vi "NI 9223 User-Controlled IO Sampling (FPGA).vi"() -> ()   [LabVIEW 2012]
doc: "This VI reads a user-defined number of points of calibrated data from all 4 channels of a NI 9223 at the specificed rate using the User-Controlled I/O Sampling API."
uses:
  <vilib>/rvi/eio/common/nirviEmuClasses.ctl
  <vilib>/rvi/eio/common/nirviEmuTemplateMethod_errors.vi
  <vilib>/rvi/Emulation/niFpgaSctlEmulationGetInTimedLoop.vi
  <vilib>/rvi/Emulation/niFpgaSctlEmulationGlobalWrite.vi
  <vilib>/rvi/interface/RandomDataEmulation/nirviRandomDataFPGAFIFO.vi
  <vilib>/rvi/interface/RandomDataEmulation/niFpgaRandomDataHandleErrors.vi
  <vilib>/eio/EIOGrowableMethodNode/genericMethod/EIOGrowableMethodNode.xnode
  <vilib>/rvi/eio/nirviEIOMethodImplementation/nirviEIOMethodImplementation.xnode
  <vilib>/rvi/eio/nirviErrorMerge/nirviErrorMerge.xnode
  <vilib>/rvi/DataTransferAndStorage/Container/XNode/niFpgaContainer.xnode
  <vilib>/rvi/interface/RandomDataEmulation/nirviRandomDataFpgaReadWriteTemplate.vi
panel:
  out "Error":bool
  in  "Number of Samples":u32=5000
  out "Error Out":errorcluster
  out "Stopped":bool
  out "Timed Out":bool
  out "Sample Gated":bool
  out "Overwrite":bool
  in  "Sample Period (uSec)":u32=1
  # "For instructions, and select Help>>Show Context Help and hover over the icon."
  # "Input Parameters"
  # "Status Information"
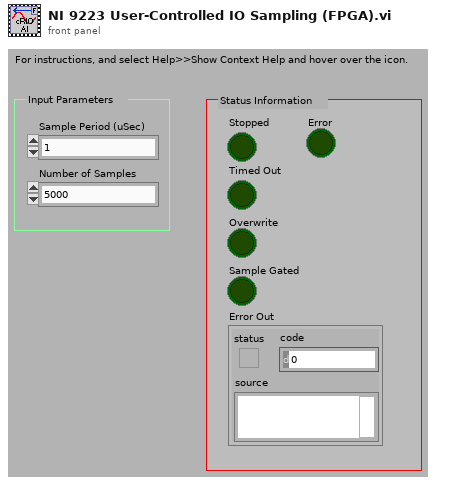
[diagram p1: front panel]
types:
  T1 = typedef "nirviEmuClasses.ctl" = enum16{"IO Read", "IO Write", "Method", "Property Read", "Property Write"}
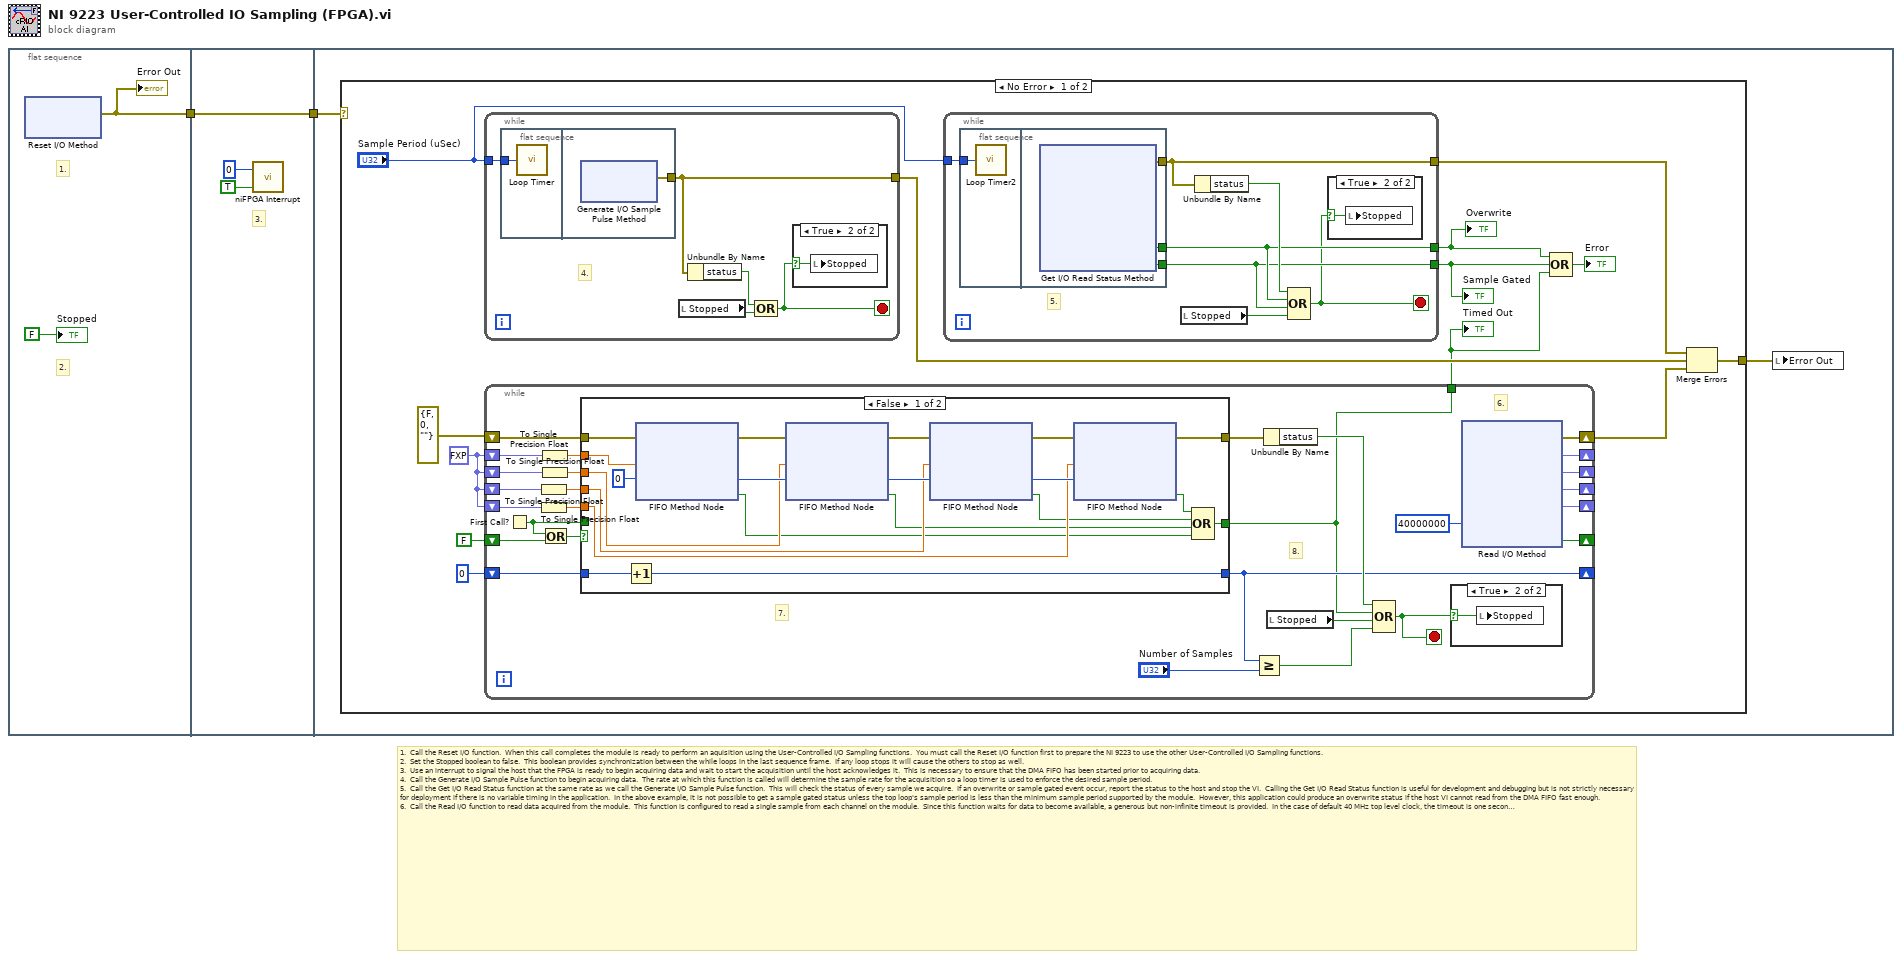
[diagram p0: block diagram]
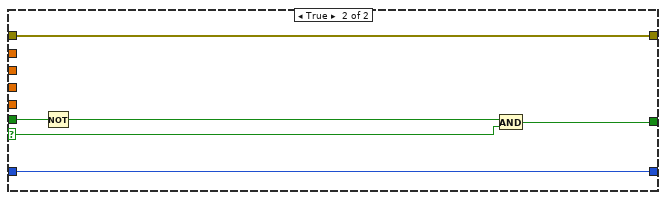
[diagram p3: hidden frame]
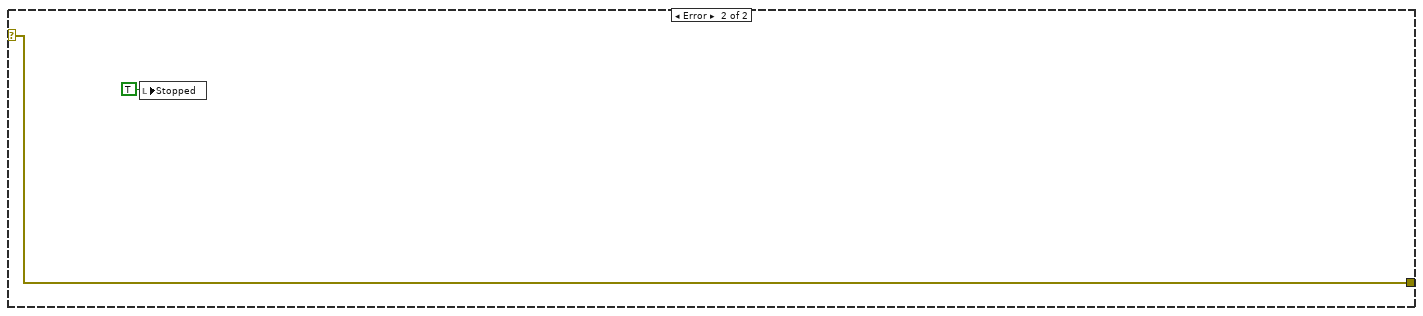
[diagram p6: hidden frame]
diagram:
  # "1.  Call the Reset I/O function.  When this call completes the module is ready to perform an aquisition using the User-Controlled I/O Sampling functions.  You must call the Reset I/O function first to prepare the NI 9223 to use the other User-Controlled I/O Sampling functions.\n2.  Set the Stopped boolean to false.  This boolean provides synchronization between the while loops in the last sequence frame.  If any loop stops it will cause the others to stop as well.\n3.  Use an interrupt to signal the host that the FPGA is ready to begin acquiring data and wait to start the acquisition until the host acknowledges it.  This is necessary to ensure that the DMA FIFO has been started prior to acquiring data.\n4.  Call the Generate I/O Sample Pulse function to begin acquiring data.  The rate at which this function is called will determine the sample rate for the acquisition so a loop timer is used to enforce the desired sample period.\n5.  Call the Get I/O Read Status function at the same rate as we call the Generate I/O Sample Pulse function.  This will check the status of every sample we acquire.  If an overwrite or sample gated event occur, report the status to the host and stop the VI.  Calling the Get I/O Read Status function is useful for development and debugging but is not strictly necessary for deployment if there is no variable timing in the application.  In the above example, it is not possible to get a sample gated status unless the top loop's sample period is less than the minimum sample period supported by the module.  However, this application could produce an overwrite status if the host VI cannot read from the DMA FIFO fast enough.\n6.  Call the Read I/O function to read data acquired from the module.  This function is configured to read a single sample from each channel on the module.  Since this function waits for data to become available, a generous but non-infinite timeout is provided.  In the case of default 40 MHz top level clock, the timeout is one second.  The acquisition loop is pipelined in order to complete each iteration quickly enough to keep up with the 1 MS/s maximum rate of the NI 9223 module.  For this reason, the data read in is immediately passed into a shift register and placed into the DMA FIFO the next iteration.\n7.  Write the acquired data into the DMA FIFO.  The FIFO Write method would normally be placed in a loop but a loop in LabVIEW FPGA adds overhead and each iteration adds two ticks to the amount of time for it to complete.  In order to complete each iteration of the while loop quickly enough to keep up with the 1 MS/s maximum rate of the NI 9223 module, this example removes the overhead of an additional loop by using a sequence of FIFO Write methods.\n8.  If a timeout occurred either while waiting for data from the module or waiting to write the data to the DMA FIFO then report the timeout to the host and stop the VI.  Otherwise stop for an error or if all requested samples have been acquired and placed into the DMA FIFO."
  n1 = flat-sequence {
    tunnel: [w3] -> w2
    tunnel: w2 -> [w50]
    tunnel: [w50] -> w1
    tunnel: w1 -> [w54]
    frame #0 {
      # "2."
      # "1."
      n2 = xnode "Reset I/O Method"() -> ("error out"=w3:errorcluster)  [unwired: 2 in, 1 out]
      "Error Out" <- w3
      "Stopped" <- FALSE ("Stopped")
    }
    frame #1 {
      # "3."
      n3 = call <vilib>:"niFPGA Interrupt.vi"("Wait Until Cleared (F)"=TRUE ("Wait Until Cleared"), "IRQ Number (0)"=u8 0 ("IRQ Number")) -> ()  [unwired: 1 in]
    }
    frame #2 {
      n4 = case shown="No Error" w54 {
        selector: w54 -> [_ w541]
        tunnel: [w67 w541] -> w53
        frame No Error {
          w65 = fxp<+/-,24,5> 0.0 ("Mod1/AI0")
          n5 = while {
            tunnel: "Sample Period (uSec)" -> [w492]
            tunnel: [w489] -> w60
            stop <- w488 stop-if-true
            # "4."
            n6 = flat-sequence {
              tunnel: w492 -> [w494]
              tunnel: [w495] -> w489
              frame #0 {
                n7 = call "Loop Timer"("Count(uSec)"=w494) -> ()  [unwired: 1 out]
              }
              frame #1 {
                n8 = xnode "Generate I/O Sample Pulse Method"() -> ("error out"=w495:errorcluster)  [unwired: 2 in, 1 out]
              }
            }
            n9 = local read "Stopped"() -> (w491:bool)
            n10 = Unbundle By Name(w489) -> ("status"=w490:bool)
            n11 = Compound Arithmetic op=OR(w490, w491) -> (w488:bool)
            n12 = case shown="True" w488 {
              selector: w488 -> [_ w493]
              frame False {
              }
              frame True {
                n13 = local write "Stopped"(w493) -> ()
              }
            }
          }
          n14 = while {
            shift-right: [w84] -> _
            shift-left: FALSE ("Timed Out") -> [w76]
            shift-right: [w79] -> w64
            shift-left: errorcluster {"status"=FALSE, "code"=0, "source"=""} ("error out") -> [w93]
            shift-right: [w80] -> _
            shift-left: w65 -> [w92]
            shift-right: [w81] -> _
            shift-left: w65 -> [w91]
            shift-right: [w82] -> _
            shift-left: w65 -> [w71]
            shift-right: [w83] -> _
            shift-left: w65 -> [w68]
            shift-right: [w86] -> _
            shift-left: u32 0 ("Number of Samples") -> [w87]
            tunnel: [w78] -> w57
            stop <- w89 stop-if-true
            # "6."
            # "7."
            # "8."
            n15 = First Call?() -> (First Call?: T/F=w74:bool)
            n16 = To Single Precision Float(number=w71) -> (single precision float=w70:sgl)
            n17 = To Single Precision Float(number=w68) -> (single precision float=w69:sgl)
            n18 = To Single Precision Float(number=w92) -> (single precision float=w73:sgl)
            n19 = To Single Precision Float(number=w91) -> (single precision float=w72:sgl)
            n20 = Or(x=w74, y=w76) -> (x .or. y?=w77:bool)
            n21 = case shown="False" w77 {
              selector: w77 -> [_ w299]
              tunnel: [w294 w303] -> w95
              tunnel: [w295 w298] -> w78
              tunnel: w93 -> [w297 w303]
              tunnel: w73 -> [w296 _]
              tunnel: w72 -> [w286 _]
              tunnel: w70 -> [w287 _]
              tunnel: w69 -> [w288 _]
              tunnel: w87 -> [w282 w302]
              tunnel: [w281 w302] -> w86
              tunnel: w74 -> [_ w301]
              frame False {
                w289 = 0 ("Timeout")
                n22 = Increment(x=w282) -> (x+1=w281:u32)
                n23 = xnode ("FIFO Method Node")("Element"=w296, "Timeout"=w289, "error in (no error)"=w297) -> ("Timed Out?"=w283:bool, "error out"=w293:errorcluster)  [unwired: 1 in, 1 out]
                n24 = xnode ("FIFO Method Node")("Element"=w286, "Timeout"=w289, "error in (no error)"=w293) -> ("Timed Out?"=w284:bool, "error out"=w292:errorcluster)  [unwired: 1 in, 1 out]
                n25 = xnode ("FIFO Method Node")("Element"=w287, "Timeout"=w289, "error in (no error)"=w292) -> ("Timed Out?"=w285:bool, "error out"=w291:errorcluster)  [unwired: 1 in, 1 out]
                n26 = xnode ("FIFO Method Node")("Element"=w288, "Timeout"=w289, "error in (no error)"=w291) -> ("Timed Out?"=w290:bool, "error out"=w294:errorcluster)  [unwired: 1 in, 1 out]
                n27 = Compound Arithmetic op=OR(w290, w285, w284, w283) -> (w295:bool)
              }
              frame True {
                n28 = Not(x=w301) -> (.not. x?=w300:bool)
                n29 = And(x=w300, y=w299) -> (x .and. y?=w298:bool)
              }
            }
            n30 = Greater Or Equal?(x=w86, y="Number of Samples") -> (x >= y?=w88:bool)
            n31 = Unbundle By Name(w95) -> ("status"=w94:bool)
            n32 = local read "Stopped"() -> (w90:bool)
            n33 = Compound Arithmetic op=OR(w94, w78, w90, w88) -> (w89:bool)
            n34 = case shown="True" w89 {
              selector: w89 -> [_ w280]
              frame False {
              }
              frame True {
                n35 = local write "Stopped"(w280) -> ()
              }
            }
            n36 = xnode "Read I/O Method"("Timeout"=40000000) -> ("error out"=w79:errorcluster, "Mod2/AI0"=w80:fxp<+/-,24,5>, "Mod2/AI1"=w81:fxp<+/-,24,5>, "Mod2/AI2"=w82:fxp<+/-,24,5>, "Mod2/AI3"=w83:fxp<+/-,24,5>, "Timed Out"=w84:bool)  [unwired: 5 in, 4 out]
          }
          "Timed Out" <- w57
          n37 = while {
            tunnel: [w310] -> w59
            tunnel: "Sample Period (uSec)" -> [w309]
            tunnel: [w306] -> w58
            tunnel: [w305] -> w56
            stop <- w304 stop-if-true
            # "5."
            n38 = flat-sequence {
              tunnel: w309 -> [w312]
              tunnel: [w315] -> w310
              tunnel: [w314] -> w306
              tunnel: [w313] -> w305
              frame #0 {
                n39 = call "Loop Timer2"("Count(uSec)"=w312) -> ()  [unwired: 1 out]
              }
              frame #1 {
                n40 = xnode "Get I/O Read Status Method"() -> ("error out"=w315:errorcluster, "Overwrite"=w314:bool, "Sample Gated"=w313:bool)  [unwired: 5 in, 4 out]
              }
            }
            n41 = local read "Stopped"() -> (w308:bool)
            n42 = Unbundle By Name(w310) -> ("status"=w307:bool)
            n43 = Compound Arithmetic op=OR(w307, w306, w305, w308) -> (w304:bool)
            n44 = case shown="True" w304 {
              selector: w304 -> [_ w311]
              frame False {
              }
              frame True {
                n45 = local write "Stopped"(w311) -> ()
              }
            }
          }
          "Overwrite" <- w58
          "Sample Gated" <- w56
          n46 = Compound Arithmetic op=OR(w58, w56, w57) -> (→"Error":bool)
          n47 = Merge Errors(w59, w60, w64) -> (w67:errorcluster)
        }
        frame Error {
          n48 = local write "Stopped"(TRUE ("Stopped")) -> ()
        }
      }
      n49 = local write "Error Out"(w53) -> ()
    }
  }
